vi "2P_AdapUprite_Linlin.vi"() -> ()   [LabVIEW 2015] (continued)
              frame True {
                n2515 = local read "wavelength(nm)"() -> (w5844:dbl)
                n2516 = call "pockelscellcalibration.vi"("l"=w5844, "T"=w5845) -> ("Vout"=w5843:dbl)
                n2517 = call "configuration_2P_Linlin.vi"("command"="get") -> ("config out"=w5841:T14)  [unwired: 2 in, 1 out]
                n2518 = Unbundle By Name(w5841) -> ("Vto2P"=w5848:i32, "AOlines"=w5847:tag[])
                n2519 = local write "Vpockels"(w5843) -> ()
                n2520 = property on="Laserpower  (%)" class="Slide (strict)"("Value"=w5845) -> ()  [unwired: 2 in, 2 out]
                n2521 = Index Array(array=w5847, index=w5848) -> (element=w5846:tag)
                n2522 = call-poly <vilib>:"DAQmx Create Virtual Channel.vi"("physical channels"=w5846) -> ("task out"=w5850:refnum<k21>, "error out"=w5849:errorcluster)  [unwired: 13 in]
                n2523 = call-poly <vilib>:"DAQmx Write.vi"("task/channels in"=w5850, "data"=w5843, "error in"=w5849) -> ("task out"=w5851:refnum<k21>, "error out"=w5852:errorcluster)  [unwired: 10 in, 1 out]
                n2524 = call <vilib>:"DAQmx Start Task.vi"("task/channels in"=w5851, "error in"=w5852) -> ("task out"=w5853:refnum<k21>, "error out"=w5854:errorcluster)  [unwired: 12 in]
                n2525 = call <vilib>:"DAQmx Stop Task.vi"("task/channels in"=w5853, "error in"=w5854) -> ("task out"=w5855:refnum<k21>, "error out"=w5856:errorcluster)  [unwired: 12 in]
                n2526 = call <vilib>:"DAQmx Clear Task.vi"("task in"=w5855, "error in"=w5856) -> ()  [unwired: 13 in, 1 out]
              }
            }
          }
          event "sealtest": Value Change {
            n2527 = event-data() -> ()  [unwired: 1 in, 6 out]
            n2528 = case shown="True" "sealtest" {
              frame False {
              }
              frame True {
                n2529 = stacked-sequence {
                  seq-local: [w5858 _ _ _ _ _ _] -> [_ w5893 _ w5945 _ _ _]
                  frame #0 {
                    n2530 = stacked-sequence {
                      tunnel: [_ w5872 _] -> w5858
                      frame #0 {
                        n2531 = call "2pparameters.vi"("command"="get") -> ("params out"=w5864:T12)  [unwired: 1 in]
                        n2532 = Unbundle By Name(w5864) -> ("autoshutter"=w5865:bool, "aAS"=w5859:u32[])
                        n2533 = local read "OCchecked?"() -> (w5862:bool)
                        n2534 = call "sealtestwfparams.vi"("command"="set") -> ()  [unwired: 6 in, 1 out]
                        n2535 = case shown="False" w5862 {
                          frame False {
                            n2536 = One Button Dialog(message="Is the OC gain correct?", button name ("OK")="ok") -> (true=w5866:bool)
                            n2537 = local write "OCchecked?"(w5866) -> ()
                          }
                          frame True {
                          }
                        }
                        n2538 = case shown="True" w5865 {
                          tunnel: w5859 -> [_ w5869]
                          frame False {
                          }
                          frame True {
                            n2539 = call "shuttercontrol_multi.vi"("Autoshutter Chans"=w5869, "command"="close") -> ()  [unwired: 1 in, 1 out]
                          }
                        }
                        n2540 = call "allAI-temp.vi"("command"=enum16{"get", "set", "clear", "append"}."clear") -> ()  [unwired: 3 in, 2 out]
                      }
                      frame #1 {
                        n2541 = call "sealtestwfparams.vi"("command"="get") -> ("Params out"=w5878:T25)  [unwired: 6 in]
                        n2542 = Unbundle By Name(w5878) -> ("AO parameters"=w5876:T26)
                        n2543 = Index Array(array=w5876, index=0) -> (element=w5875:T27)
                        n2544 = call "generateRampedSquareWave_fromAOparameters.vi"("AO params"=w5875) -> ("Waveform"=w5871:waveform(dbl), "wflength"=w5872:i32)
                        n2545 = Build Array(w5871) -> (w5874:waveform(dbl)[])
                        n2546 = call "waveformssealtestbuffer.vi"("AO wf in"=w5874, "command"="set") -> ()  [unwired: 1 out]
                      }
                      frame #2 {
                        n2547 = local read "Vholding (mV)"() -> (w5881:sgl)
                        n2548 = local read "Current Clamp"() -> (w5887:bool)
                        n2549 = local read "Voltage Clamp"() -> (w5886:bool)
                        n2550 = local read "OCgain"() -> (w5882:sgl)
                        n2551 = local read "CC_ICgain"() -> (w5885:dbl)
                        n2552 = local read "holdon"() -> (w5880:bool)
                        n2553 = call "patchparameters.vi"("command"="get") -> ("Params out"=w5889:T16)  [unwired: 1 in]
                        n2554 = Bundle By Name(cluster=w5889, "VC"=w5886, "CC"=w5887, "CC_icg (pA/mv)"=w5885, "VC_icg (mV/mV)"=10.0, "OCG (mV/pA)"=w5882, "OVG (mV/mV)"=0.1, "Vhold (mV)"=w5881, "holdon"=w5880) -> (w5888:T16)
                        n2555 = call "patchparameters.vi"("Params in"=w5888, "command"="set") -> ()  [unwired: 1 out]
                      }
                    }
                  }
                  frame #1 {
                    w5892 = 2
                    n2556 = call "patchparameters.vi"("command"="get") -> ("Params out"=w5900:T16)  [unwired: 1 in]
                    n2557 = Unbundle By Name(w5900) -> ("holdon"=w5899:bool, "Vhold (mV)"=w5898:sgl, "CC_icg (pA/mv)"=w5906:sgl, "CC"=w5904:bool, "VC_icg (mV/mV)"=w5905:sgl)
                    n2558 = Select(t=w5906, s=w5904, f=w5905) -> (s? t:f=w5907:sgl)
                    n2559 = To Single Precision Float(number=0.001 ("y")) -> (single precision float=w5908:sgl)
                    n2560 = Compound Arithmetic op=MULTIPLY(w5898, w5907, w5908) -> (w5902:sgl)
                    n2561 = case shown="False" w5899 {
                      tunnel: w5902 -> [_ w5920]
                      tunnel: [0.0 w5920] -> w5895
                      frame False {
                      }
                      frame True {
                      }
                    }
                    n2562 = Greater Than 0?(x=w5892) -> (x > 0?=w5894:bool)
                    n2563 = case shown="True" w5894 {
                      tunnel: w5893 -> [_ w5909]
                      tunnel: w5892 -> [_ w5912]
                      frame False {
                      }
                      frame True {
                        n2564 = Initialize Array(sgl 0.0 ("element"), w5912, w5909) -> (w5910:sgl[][])
                        n2565 = call "allAI-temp.vi"("array in"=w5910, "command"=enum16{"get", "set", "clear", "append"}."set") -> ()  [unwired: 2 in, 2 out]
                      }
                    }
                    n2566 = flat-sequence {
                      tunnel: w5893 -> [w5916]
                      tunnel: w5893 -> [w5915]
                      tunnel: [w5915] -> w5897
                      tunnel: [w5914] -> w5896
                      tunnel: w5895 -> [w5914]
                      tunnel: w5897 -> [w5918]
                      tunnel: w5896 -> [w5917]
                      frame #0 {
                        n2567 = call "prepAI_sealtest.vi"("samples per channel"=w5916) -> ()  [unwired: 2 in]
                      }
                      frame #1 {
                        n2568 = call "prepAO_sealtest.vi"("Vhold"=w5917, "samples per channel"=w5918) -> ()  [unwired: 1 in]
                      }
                    }
                  }
                  frame #2 {
                    n2569 = stacked-sequence {
                      frame #0 {
                        n2570 = call "tempconfigAO_seal.vi"("command"="get") -> ("Temp Config out"=w5924:T28)  [unwired: 1 in]
                        n2571 = Unbundle By Name(w5924) -> ("AO"=w5925:refnum<k21>[], "E_AO"=w5926:errorcluster[])
                        n2572 = for {
                          tunnel: w5925 -> [w5934] mode=indexing
                          tunnel: w5926 -> [w5933] mode=indexing
                          tunnel: [w5932] -> w5928 mode=indexing
                          tunnel: [w5931] -> w5929 mode=indexing
                          n2573 = call <vilib>:"DAQmx Start Task.vi"("task/channels in"=w5934, "error in"=w5933) -> ("task out"=w5932:refnum<k21>, "error out"=w5931:errorcluster)  [unwired: 12 in]
                        }
                        n2574 = call "tempconfigAO_seal.vi"("command"="get") -> ("Temp Config out"=w5927:T28)  [unwired: 1 in]
                        n2575 = Bundle By Name(cluster=w5927, "AO"=w5928, "E_AO"=w5929) -> (w5930:T28)
                        n2576 = call "tempconfigAO_seal.vi"("Temp Config in"=w5930, "command"="set") -> ()  [unwired: 1 out]
                      }
                      frame #1 {
                        n2577 = call "tempconfigAI_seal.vi"("command"="get") -> ("Temp Config out"=w5936:T29)  [unwired: 1 in]
                        n2578 = Unbundle By Name(w5936) -> ("AI"=w5941:refnum<k21>, "E_AI"=w5942:errorcluster)
                        n2579 = call <vilib>:"DAQmx Start Task.vi"("task/channels in"=w5941, "error in"=w5942) -> ("task out"=w5943:refnum<k21>, "error out"=w5944:errorcluster)  [unwired: 12 in]
                        n2580 = call "tempconfigAI_seal.vi"("command"="get") -> ("Temp Config out"=w5938:T29)  [unwired: 1 in]
                        n2581 = Bundle By Name(cluster=w5938, "AI"=w5943, "E_AI"=w5944) -> (w5940:T29)
                        n2582 = call "tempconfigAI_seal.vi"("Temp Config in"=w5940, "command"="set") -> ()  [unwired: 1 out]
                      }
                    }
                  }
                  frame #3 {
                    n2583 = while {
                      tunnel: w5945 -> [w5946]
                      stop <- w5947 stop-if-true
                      n2584 = stacked-sequence {
                        seq-local: [_ _ _ w5988 _ _] -> [_ _ _ _ w6040 _]
                        seq-local: [w5949 _ _ _ _ _] -> [_ w5958 _ w5981 w6029 w6060]
                        tunnel: w5946 -> [_ _ w5966 _ w6028 _]
                        frame #0 {
                          n2585 = call "patchparameters.vi"("command"="get") -> ("Params out"=w5956:T16)  [unwired: 1 in]
                          n2586 = local read "Vholding (mV)"() -> (w5953:sgl)
                          n2587 = Unbundle By Name(w5956) -> ("Vhold (mV)"=w5952:sgl, "holdon"=w5955:bool)
                          n2588 = local read "holdon"() -> (w5954:bool)
                          n2589 = Not Equal?(x=w5953, y=w5952) -> (x != y?=w5951:bool)
                          n2590 = Not Equal?(x=w5955, y=w5954) -> (x != y?=w5950:bool)
                          n2591 = Or(x=w5951, y=w5950) -> (x .or. y?=w5949:bool)
                        }
                        frame #1 {
                          n2592 = case shown="True" w5958 {
                            frame False {
                            }
                            frame True {
                              n2593 = local read "Vholding (mV)"() -> (w5961:sgl)
                              n2594 = local read "holdon"() -> (w5959:bool)
                              n2595 = call "patchparameters.vi"("command"="get") -> ("Params out"=w5962:T16)  [unwired: 1 in]
                              n2596 = Bundle By Name(cluster=w5962, "Vhold (mV)"=w5961, "holdon"=w5959) -> (w5960:T16)
                              n2597 = call "patchparameters.vi"("Params in"=w5960, "command"="set") -> ()  [unwired: 1 out]
                            }
                          }
                        }
                        frame #2 {
                          n2598 = call "tempconfigAI_seal.vi"("command"="get") -> ("Temp Config out"=w5976:T29)  [unwired: 1 in]
                          n2599 = Unbundle By Name(w5976) -> ("AI"=w5975:refnum<k21>, "E_AI"=w5974:errorcluster)
                          n2600 = call-poly <vilib>:"DAQmx Read.vi"("task/channels in"=w5975, "number of samples per channel"=w5966, "timeout"=10.0, "error in"=w5974) -> ("task out"=w5970:refnum<k21>, "data"=w5967:i16[][], "error out"=w5979:errorcluster)  [unwired: 9 in]
                          n2601 = call "tempconfigAI_seal.vi"("command"="get") -> ("Temp Config out"=w5971:T29)  [unwired: 1 in]
                          n2602 = Bundle By Name(cluster=w5971, "AI"=w5970, "E_AI"=w5979) -> (w5978:T29)
                          n2603 = To Single Precision Float(number=w5967) -> (single precision float=w5969:sgl[][])
                          n2604 = call "tempconfigAI_seal.vi"("Temp Config in"=w5978, "command"="set") -> ()  [unwired: 1 out]
                          n2605 = call "allAI-temp.vi"("array in"=w5969, "command"=enum16{"get", "set", "clear", "append"}."set") -> ()  [unwired: 2 in, 2 out]
                        }
                        frame #3 {
                          n2606 = case shown="True" w5981 {
                            frame False {
                            }
                            frame True {
                              n2607 = call "tempconfigAO_seal.vi"("command"="get") -> ("Temp Config out"=w6017:T28)  [unwired: 1 in]
                              n2608 = Unbundle By Name(w6017) -> ("AO"=w6016:refnum<k21>[], "E_AO"=w6015:errorcluster[])
                              n2609 = call "tempconfigAI_seal.vi"("command"="get") -> ("Temp Config out"=w6004:T29)  [unwired: 1 in]
                              n2610 = Unbundle By Name(w6004) -> ("AI"=w6005:refnum<k21>, "E_AI"=w6006:errorcluster)
                              n2611 = for {
                                tunnel: w6016 -> [w6021] mode=indexing
                                tunnel: w6015 -> [w6020] mode=indexing
                                tunnel: [w6019] -> w6011 mode=indexing
                                n2612 = call <vilib>:"DAQmx Stop Task.vi"("task/channels in"=w6021, "error in"=w6020) -> ("task out"=w6022:refnum<k21>, "error out"=w6023:errorcluster)  [unwired: 12 in]
                                n2613 = call <vilib>:"DAQmx Clear Task.vi"("task in"=w6022, "error in"=w6023) -> ("error out"=w6019:errorcluster)  [unwired: 13 in]
                              }
                              n2614 = call <vilib>:"DAQmx Stop Task.vi"("task/channels in"=w6005, "error in"=w6006) -> ("task out"=w6002:refnum<k21>, "error out"=w6001:errorcluster)  [unwired: 12 in]
                              n2615 = call <vilib>:"DAQmx Clear Task.vi"("task in"=w6002, "error in"=w6001) -> ("error out"=w6000:errorcluster)  [unwired: 13 in]
                              n2616 = call "tempconfigAO_seal.vi"("command"="get") -> ("Temp Config out"=w6012:T28)  [unwired: 1 in]
                              n2617 = Bundle By Name(cluster=w6012, "E_AO"=w6011) -> (w6010:T28)
                              n2618 = call "tempconfigAI_seal.vi"("command"="get") -> ("Temp Config out"=w6008:T29)  [unwired: 1 in]
                              n2619 = Bundle By Name(cluster=w6008, "E_AI"=w6000) -> (w5999:T29)
                              n2620 = call "tempconfigAO_seal.vi"("Temp Config in"=w6010, "command"="set") -> ()  [unwired: 1 out]
                              n2621 = call "tempconfigAI_seal.vi"("Temp Config in"=w5999, "command"="set") -> ()  [unwired: 1 out]
                            }
                          }
                          n2622 = call "allAI-temp.vi"("command"=enum16{"get", "set", "clear", "append"}."get") -> ("array out"=w5985:sgl[][])  [unwired: 3 in, 1 out]
                          n2623 = call "tempconfigAI_seal.vi"("command"="get") -> ("Temp Config out"=w5997:T29)  [unwired: 1 in]
                          n2624 = Unbundle By Name(w5997) -> ("header"=w5980:dbl[])
                          n2625 = Index Array(array=w5985, index (row) #1=1 ("index (row)"), index (row) #2=0 ("index (row)")) -> (element #1=w5983:sgl[], element #2=w5982:sgl[])  [unwired: 2 in]
                          n2626 = local read "OCgain"() -> (w5990:sgl)
                          n2627 = call "Unscaledtoscaled.vi"("Unscaled Data"=w5983, "Header Information"=w5980) -> ("Array"=w5995:sgl[])  [unwired: 1 in]
                          n2628 = call "Unscaledtoscaled.vi"("Unscaled Data"=w5982, "Header Information"=w5980) -> ("Array"=w5998:sgl[])  [unwired: 1 in]
                          n2629 = Multiply(x=w5995, y=0.1) -> (x*y=w5992:dbl[])
                          n2630 = Divide(x=w5998, y=w5990) -> (x/y=w5991:sgl[])
                          n2631 = Build Array(w5992, w5991) -> (w5994:dbl[][])
                          n2632 = Multiply(x=w5994, y=1000.0) -> (x*y=w5988:dbl[][])
                          "Patch readout" <- w5988
                        }
                        frame #4 {
                          n2633 = case shown="True" w6029 {
                            tunnel: w6028 -> [_ w6041]
                            frame False {
                            }
                            frame True {
                              n2634 = call "patchparameters.vi"("command"="get") -> ("Params out"=w6045:T16)  [unwired: 1 in]
                              n2635 = Unbundle By Name(w6045) -> ("holdon"=w6044:bool, "Vhold (mV)"=w6043:sgl, "CC_icg (pA/mv)"=w6051:sgl, "CC"=w6049:bool, "VC_icg (mV/mV)"=w6050:sgl)
                              n2636 = Select(t=w6051, s=w6049, f=w6050) -> (s? t:f=w6052:sgl)
                              n2637 = To Single Precision Float(number=0.001 ("y")) -> (single precision float=w6053:sgl)
                              n2638 = Compound Arithmetic op=MULTIPLY(w6043, w6052, w6053) -> (w6047:sgl)
                              n2639 = case shown="True" w6044 {
                                tunnel: w6047 -> [_ w6058]
                                tunnel: [0.0 w6058] -> w6042
                                frame False {
                                }
                                frame True {
                                }
                              }
                              n2640 = flat-sequence {
                                tunnel: w6041 -> [w6054]
                                tunnel: w6042 -> [w6056]
                                tunnel: w6041 -> [w6055]
                                frame #0 {
                                n2641 = call "prepAI_sealtest.vi"("samples per channel"=w6054) -> ()  [unwired: 2 in]
                                }
                                frame #1 {
                                n2642 = call "prepAO_sealtest.vi"("Vhold"=w6056, "samples per channel"=w6055) -> ()  [unwired: 1 in]
                                }
                              }
                            }
                          }
                          n2643 = call "sealtestwfparams.vi"("command"="get") -> ("Params out"=w6034:T25)  [unwired: 6 in]
                          n2644 = Unbundle By Name(w6034) -> ("AO parameters"=w6035:T26)
                          n2645 = Index Array(array=w6035, index=0) -> (element=w6037:T27)
                          n2646 = Unbundle By Name(w6037) -> ("Cycles"=w6032:dbl, "Start amplitude (V)"=w6031:dbl, "Sampling frequency (Hz)"=w6030:dbl)
                          n2647 = local read "fitpoints"() -> (w6038:dbl)
                          n2648 = script code="V=data(1,:);\nI=data(2,:);\ntres=mean(V);\nspc=(nsamp./ncyc);\nV=V(spc+1:end-spc);\nI=I(spc+1:end-spc);\ndV=mean(V(V>tres))-mean(V(V<tres))\nIcyc=reshape(I,[spc ncyc-2]);\nIcyc=Icyc';\nIcyc=mean(Icyc,1);\ndIss=mean(Icyc(floor(spc*0.15):floor(spc/2)-2))-mean(Icyc(spc*0.65:spc-2))\nRm=dV*1e3/dIss;\n[maxi,ind]=max(Icyc);\nIfit=Icyc(ind+1:ind+1+points-1)-0.5*(mean(Icyc(floor(spc*0.15):floor(spc/2)-2))+mean(Icyc(spc*0.65:spc-2)))\nt=(3:points-1+3)./srate*1000;\nt=t';\nIfit=Ifit';\nc=fit(t,Ifit, 'exp1');\ncoeffs=coeffvalues(c);\nIa=coeffs(1);\nRa=dV*1e3./Ia/2;\ntau=-1./coeffs(2);\ncap=tau/Ra*1000;"("data"=w6040, "nsamp"=w6028, "ncyc"=w6032, "maxV"=w6031, "points"=w6038, "srate"=w6030) -> ("cap"=w6027:dbl, "Ra"=w6026:dbl, "Icyc"=w6025:dbl[], "Rm"=w6024:dbl)  [unwired: 1 in, 1 out]
                          n2649 = local read "set as Rp?"() -> (w6039:bool)
                          n2650 = local write "Cmembrane"(w6027) -> ()
                          n2651 = local write "Rmembrane (MOhm)"(w6024) -> ()
                          n2652 = local write "Racces (MOhm)"(w6026) -> ()
                          n2653 = case shown="True" w6039 {
                            tunnel: w6024 -> [_ w6059]
                            frame False {
                            }
                            frame True {
                              n2654 = local write "Rpipette (MOhm)"(w6059) -> ()
                            }
                          }
                          n2655 = local write "Ifit"(w6025) -> ()
                        }
                        frame #5 {
                          n2656 = local read "set as Rp?"() -> (w6061:bool)
                          n2657 = case shown="True" w6060 {
                            frame False {
                            }
                            frame True {
                              n2658 = stacked-sequence {
                                frame #0 {
                                n2659 = call "tempconfigAO_seal.vi"("command"="get") -> ("Temp Config out"=w6068:T28)  [unwired: 1 in]
                                n2660 = Unbundle By Name(w6068) -> ("AO"=w6067:refnum<k21>[], "E_AO"=w6066:errorcluster[])
                                n2661 = for {
                                tunnel: w6067 -> [w6075] mode=indexing
                                tunnel: w6066 -> [w6074] mode=indexing
                                tunnel: [w6073] -> w6064 mode=indexing
                                tunnel: [w6072] -> w6063 mode=indexing
                                n2662 = call <vilib>:"DAQmx Start Task.vi"("task/channels in"=w6075, "error in"=w6074) -> ("task out"=w6073:refnum<k21>, "error out"=w6072:errorcluster)  [unwired: 12 in]
                                }
                                n2663 = call "tempconfigAO_seal.vi"("command"="get") -> ("Temp Config out"=w6065:T28)  [unwired: 1 in]
                                n2664 = Bundle By Name(cluster=w6065, "AO"=w6064, "E_AO"=w6063) -> (w6062:T28)
                                n2665 = call "tempconfigAO_seal.vi"("Temp Config in"=w6062, "command"="set") -> ()  [unwired: 1 out]
                                }
                                frame #1 {
                                n2666 = call "tempconfigAI_seal.vi"("command"="get") -> ("Temp Config out"=w6077:T29)  [unwired: 1 in]
                                n2667 = Unbundle By Name(w6077) -> ("AI"=w6082:refnum<k21>, "E_AI"=w6083:errorcluster)
                                n2668 = call <vilib>:"DAQmx Start Task.vi"("task/channels in"=w6082, "error in"=w6083) -> ("task out"=w6084:refnum<k21>, "error out"=w6085:errorcluster)  [unwired: 12 in]
                                n2669 = call "tempconfigAI_seal.vi"("command"="get") -> ("Temp Config out"=w6079:T29)  [unwired: 1 in]
                                n2670 = Bundle By Name(cluster=w6079, "AI"=w6084, "E_AI"=w6085) -> (w6081:T29)
                                n2671 = call "tempconfigAI_seal.vi"("Temp Config in"=w6081, "command"="set") -> ()  [unwired: 1 out]
                                }
                              }
                            }
                          }
                          n2672 = case shown="True" w6061 {
                            frame False {
                            }
                            frame True {
                              n2673 = local write "set as Rp?"(FALSE ("set as Rp?")) -> ()
                            }
                          }
                        }
                      }
                      n2674 = local read "sealtest"() -> (w5948:bool)
                      n2675 = Not(x=w5948) -> (.not. x?=w5947:bool)
                    }
                  }
                  frame #4 {
                    n2676 = call "tempconfigAO_seal.vi"("command"="get") -> ("Temp Config out"=w6112:T28)  [unwired: 1 in]
                    n2677 = call "configuration_2P_Linlin.vi"("command"="get") -> ("config out"=w6087:T14)  [unwired: 2 in, 1 out]
                    n2678 = Unbundle By Name(w6112) -> ("AO"=w6111:refnum<k21>[], "E_AO"=w6110:errorcluster[])
                    n2679 = call "tempconfigAI_seal.vi"("command"="get") -> ("Temp Config out"=w6099:T29)  [unwired: 1 in]
                    n2680 = Unbundle By Name(w6099) -> ("AI"=w6100:refnum<k21>, "E_AI"=w6101:errorcluster)
                    n2681 = Unbundle By Name(w6087) -> ("Device 1 sampleclock out"=w6092:tag, "Device 1 Starttrigger out"=w6091:tag)
                    n2682 = for {
                      tunnel: w6111 -> [w6116] mode=indexing
                      tunnel: w6110 -> [w6115] mode=indexing
                      tunnel: [w6114] -> w6106 mode=indexing
                      n2683 = call <vilib>:"DAQmx Stop Task.vi"("task/channels in"=w6116, "error in"=w6115) -> ("task out"=w6117:refnum<k21>, "error out"=w6118:errorcluster)  [unwired: 12 in]
                      n2684 = call <vilib>:"DAQmx Clear Task.vi"("task in"=w6117, "error in"=w6118) -> ("error out"=w6114:errorcluster)  [unwired: 13 in]
                    }
                    n2685 = call <vilib>:"DAQmx Stop Task.vi"("task/channels in"=w6100, "error in"=w6101) -> ("task out"=w6097:refnum<k21>, "error out"=w6096:errorcluster)  [unwired: 12 in]
                    n2686 = call <vilib>:"DAQmx Disconnect Terminals.vi"("source terminal"=tag "/Dev1/ai/SampleClock", "destination terminal"=w6092) -> ("error out"=w6089:errorcluster)  [unwired: 13 in]
                    n2687 = call <vilib>:"DAQmx Clear Task.vi"("task in"=w6097, "error in"=w6096) -> ("error out"=w6095:errorcluster)  [unwired: 13 in]
                    n2688 = call "tempconfigAO_seal.vi"("command"="get") -> ("Temp Config out"=w6107:T28)  [unwired: 1 in]
                    n2689 = Bundle By Name(cluster=w6107, "E_AO"=w6106) -> (w6105:T28)
                    n2690 = call "tempconfigAI_seal.vi"("command"="get") -> ("Temp Config out"=w6103:T29)  [unwired: 1 in]
                    n2691 = Bundle By Name(cluster=w6103, "E_AI"=w6095) -> (w6094:T29)
                    n2692 = call "tempconfigAO_seal.vi"("Temp Config in"=w6105, "command"="set") -> ()  [unwired: 1 out]
                    n2693 = call "tempconfigAI_seal.vi"("Temp Config in"=w6094, "command"="set") -> ()  [unwired: 1 out]
                    n2694 = call <vilib>:"DAQmx Disconnect Terminals.vi"("source terminal"=tag "/Dev1/ai/StartTrigger", "destination terminal"=w6091, "error in"=w6089) -> ()  [unwired: 12 in, 1 out]
                  }
                  frame #5 {
                    n2695 = call "zeropatch.vi"() -> ()  [unwired: 12 in]
                  }
                  frame #6 {
                    w6122 = T24 4 items=["no dialog", "OK message", "continue or stop message", "OK message + warnings", "continue/stop + warnings"] ("type of dialog (OK msg:1)")
                    n2696 = call "displayerrors.vi"() -> ("error IO"=w6121:errorcluster)
                    n2697 = call <vilib>:"Simple Error Handler.vi"("type of dialog (OK msg:1)"=w6122, "error in (no error)"=w6121) -> ("error out"=w6120:errorcluster)  [unwired: 3 in, 4 out]
                    n2698 = call <vilib>:"Clear Errors.vi"("error in (no error)"=w6120) -> ("error out"=w6119:errorcluster)  [unwired: 5 in, 1 out]
                    n2699 = call "seterrors.vi"("error IO"=w6119) -> ()
                  }
                }
              }
            }
          }
          event "readpatch": Value Change {
            n2700 = event-data() -> ()  [unwired: 1 in, 6 out]
            n2701 = local read "readpatch"() -> (w6123:bool)
            n2702 = case shown="True" w6123 {
              frame False {
              }
              frame True {
                n2703 = stacked-sequence {
                  seq-local: [w6124 _ _ _ _ _] -> [_ w6159 _ w6211 _ _]
                  frame #0 {
                    n2704 = stacked-sequence {
                      tunnel: [_ w6138 _] -> w6124
                      frame #0 {
                        n2705 = call "2pparameters.vi"("command"="get") -> ("params out"=w6130:T12)  [unwired: 1 in]
                        n2706 = Unbundle By Name(w6130) -> ("autoshutter"=w6131:bool, "aAS"=w6125:u32[])
                        n2707 = local read "OCchecked?"() -> (w6128:bool)
                        n2708 = call "sealtestwfparams.vi"("command"="set") -> ()  [unwired: 6 in, 1 out]
                        n2709 = case shown="False" w6128 {
                          frame False {
                            n2710 = One Button Dialog(message="Is the OC gain correct?", button name ("OK")="ok") -> (true=w6132:bool)
                            n2711 = local write "OCchecked?"(w6132) -> ()
                          }
                          frame True {
                          }
                        }
                        n2712 = case shown="True" w6131 {
                          tunnel: w6125 -> [_ w6135]
                          frame False {
                          }
                          frame True {
                            n2713 = call "shuttercontrol_multi.vi"("Autoshutter Chans"=w6135, "command"="close") -> ()  [unwired: 1 in, 1 out]
                          }
                        }
                        n2714 = call "allAI-temp.vi"("command"=enum16{"get", "set", "clear", "append"}."clear") -> ()  [unwired: 3 in, 2 out]
                      }
                      frame #1 {
                        n2715 = call "sealtestwfparams.vi"("command"="get") -> ("Params out"=w6144:T25)  [unwired: 6 in]
                        n2716 = Unbundle By Name(w6144) -> ("AO parameters"=w6142:T26)
                        n2717 = Index Array(array=w6142, index=1) -> (element=w6141:T27)
                        n2718 = call "generateRampedSquareWave_fromAOparameters.vi"("AO params"=w6141) -> ("Waveform"=w6137:waveform(dbl), "wflength"=w6138:i32)
                        n2719 = Build Array(w6137) -> (w6140:waveform(dbl)[])
                        n2720 = call "waveformssealtestbuffer.vi"("AO wf in"=w6140, "command"="set") -> ()  [unwired: 1 out]
                      }
                      frame #2 {
                        n2721 = local read "Vholding (mV)"() -> (w6147:sgl)
                        n2722 = local read "Current Clamp"() -> (w6153:bool)
                        n2723 = local read "Voltage Clamp"() -> (w6152:bool)
                        n2724 = local read "OCgain"() -> (w6148:sgl)
                        n2725 = local read "CC_ICgain"() -> (w6151:dbl)
                        n2726 = local read "holdon"() -> (w6146:bool)
                        n2727 = call "patchparameters.vi"("command"="get") -> ("Params out"=w6155:T16)  [unwired: 1 in]
                        n2728 = Bundle By Name(cluster=w6155, "VC"=w6152, "CC"=w6153, "CC_icg (pA/mv)"=w6151, "VC_icg (mV/mV)"=10.0, "OCG (mV/pA)"=w6148, "OVG (mV/mV)"=0.1, "Vhold (mV)"=w6147, "holdon"=w6146) -> (w6154:T16)
                        n2729 = call "patchparameters.vi"("Params in"=w6154, "command"="set") -> ()  [unwired: 1 out]
                      }
                    }
                  }
                  frame #1 {
                    w6158 = 2
                    n2730 = call "patchparameters.vi"("command"="get") -> ("Params out"=w6166:T16)  [unwired: 1 in]
                    n2731 = Unbundle By Name(w6166) -> ("holdon"=w6165:bool, "Vhold (mV)"=w6164:sgl, "CC_icg (pA/mv)"=w6172:sgl, "CC"=w6170:bool, "VC_icg (mV/mV)"=w6171:sgl)
                    n2732 = Select(t=w6172, s=w6170, f=w6171) -> (s? t:f=w6173:sgl)
                    n2733 = To Single Precision Float(number=0.001 ("y")) -> (single precision float=w6174:sgl)
                    n2734 = Compound Arithmetic op=MULTIPLY(w6164, w6173, w6174) -> (w6168:sgl)
                    n2735 = case shown="False" w6165 {
                      tunnel: w6168 -> [_ w6186]
                      tunnel: [0.0 w6186] -> w6161
                      frame False {
                      }
                      frame True {
                      }
                    }
                    n2736 = Greater Than 0?(x=w6158) -> (x > 0?=w6160:bool)
                    n2737 = case shown="True" w6160 {
                      tunnel: w6159 -> [_ w6175]
                      tunnel: w6158 -> [_ w6178]
                      frame False {
                      }
                      frame True {
                        n2738 = Initialize Array(sgl 0.0 ("element"), w6178, w6175) -> (w6176:sgl[][])
                        n2739 = call "allAI-temp.vi"("array in"=w6176, "command"=enum16{"get", "set", "clear", "append"}."set") -> ()  [unwired: 2 in, 2 out]
                      }
                    }
                    n2740 = flat-sequence {
                      tunnel: w6159 -> [w6182]
                      tunnel: w6159 -> [w6181]
                      tunnel: [w6181] -> w6163
                      tunnel: [w6180] -> w6162
                      tunnel: w6161 -> [w6180]
                      tunnel: w6163 -> [w6184]
                      tunnel: w6162 -> [w6183]
                      frame #0 {
                        n2741 = call "prepAI_sealtest.vi"("samples per channel"=w6182) -> ()  [unwired: 2 in]
                      }
                      frame #1 {
                        n2742 = call "prepAO_sealtest.vi"("Vhold"=w6183, "samples per channel"=w6184) -> ()  [unwired: 1 in]
                      }
                    }
                  }
                  frame #2 {
                    n2743 = stacked-sequence {
                      frame #0 {
                        n2744 = call "tempconfigAO.vi"("command"="get") -> ("Temp Config out"=w6190:T28)  [unwired: 1 in]
                        n2745 = Unbundle By Name(w6190) -> ("AO"=w6191:refnum<k21>[], "E_AO"=w6192:errorcluster[])
                        n2746 = for {
                          tunnel: w6191 -> [w6200] mode=indexing
                          tunnel: w6192 -> [w6199] mode=indexing
                          tunnel: [w6198] -> w6194 mode=indexing
                          tunnel: [w6197] -> w6195 mode=indexing
                          n2747 = call <vilib>:"DAQmx Start Task.vi"("task/channels in"=w6200, "error in"=w6199) -> ("task out"=w6198:refnum<k21>, "error out"=w6197:errorcluster)  [unwired: 12 in]
                        }
                        n2748 = call "tempconfigAO.vi"("command"="get") -> ("Temp Config out"=w6193:T28)  [unwired: 1 in]
                        n2749 = Bundle By Name(cluster=w6193, "AO"=w6194, "E_AO"=w6195) -> (w6196:T28)
                        n2750 = call "tempconfigAO.vi"("Temp Config in"=w6196, "command"="set") -> ()  [unwired: 1 out]
                      }
                      frame #1 {
                        n2751 = call "tempconfigAI.vi"("command"="get") -> ("Temp Config out"=w6202:T29)  [unwired: 1 in]
                        n2752 = Unbundle By Name(w6202) -> ("AI"=w6207:refnum<k21>, "E_AI"=w6208:errorcluster)
                        n2753 = call <vilib>:"DAQmx Start Task.vi"("task/channels in"=w6207, "error in"=w6208) -> ("task out"=w6209:refnum<k21>, "error out"=w6210:errorcluster)  [unwired: 12 in]
                        n2754 = call "tempconfigAI.vi"("command"="get") -> ("Temp Config out"=w6204:T29)  [unwired: 1 in]
                        n2755 = Bundle By Name(cluster=w6204, "AI"=w6209, "E_AI"=w6210) -> (w6206:T29)
                        n2756 = call "tempconfigAI.vi"("Temp Config in"=w6206, "command"="set") -> ()  [unwired: 1 out]
                      }
                    }
                  }
                  frame #3 {
                    n2757 = while {
                      tunnel: w6211 -> [w6212]
                      stop <- w6213 stop-if-true
                      n2758 = local read "readpatch"() -> (w6216:bool)
                      n2759 = Not(x=w6216) -> (.not. x?=w6215:bool)
                      n2760 = case shown="False" w6215 {
                        tunnel: w6212 -> [w6217 _]
                        frame False {
                          n2761 = stacked-sequence {
                            seq-local: [w6218 _ _ _ _ _] -> [_ w6227 _ w6250 w6297 w6316]
                            tunnel: w6217 -> [_ _ w6235 _ w6296 _]
                            frame #0 {
                              n2762 = call "patchparameters.vi"("command"="get") -> ("Params out"=w6225:T16)  [unwired: 1 in]
                              n2763 = local read "Vholding (mV)"() -> (w6222:sgl)
                              n2764 = Unbundle By Name(w6225) -> ("Vhold (mV)"=w6221:sgl, "holdon"=w6224:bool)
                              n2765 = local read "holdon"() -> (w6223:bool)
                              n2766 = Not Equal?(x=w6222, y=w6221) -> (x != y?=w6220:bool)
                              n2767 = Not Equal?(x=w6224, y=w6223) -> (x != y?=w6219:bool)
                              n2768 = Or(x=w6220, y=w6219) -> (x .or. y?=w6218:bool)
                            }
                            frame #1 {
                              n2769 = case shown="False" w6227 {
                                frame False {
                                }
                                frame True {
                                n2770 = local read "Vholding (mV)"() -> (w6230:sgl)
                                n2771 = local read "holdon"() -> (w6228:bool)
                                n2772 = call "patchparameters.vi"("command"="get") -> ("Params out"=w6231:T16)  [unwired: 1 in]
                                n2773 = Bundle By Name(cluster=w6231, "Vhold (mV)"=w6230, "holdon"=w6228) -> (w6229:T16)
                                n2774 = call "patchparameters.vi"("Params in"=w6229, "command"="set") -> ()  [unwired: 1 out]
                                }
                              }
                            }
                            frame #2 {
                              n2775 = call "tempconfigAI.vi"("command"="get") -> ("Temp Config out"=w6245:T29)  [unwired: 1 in]
                              n2776 = Unbundle By Name(w6245) -> ("AI"=w6244:refnum<k21>, "E_AI"=w6243:errorcluster)
                              n2777 = call-poly <vilib>:"DAQmx Read.vi"("task/channels in"=w6244, "number of samples per channel"=w6235, "timeout"=10.0, "error in"=w6243) -> ("task out"=w6239:refnum<k21>, "data"=w6236:i16[][], "error out"=w6248:errorcluster)  [unwired: 9 in]
                              n2778 = call "tempconfigAI.vi"("command"="get") -> ("Temp Config out"=w6240:T29)  [unwired: 1 in]
                              n2779 = Bundle By Name(cluster=w6240, "AI"=w6239, "E_AI"=w6248) -> (w6247:T29)
                              n2780 = To Single Precision Float(number=w6236) -> (single precision float=w6238:sgl[][])
                              n2781 = call "tempconfigAI.vi"("Temp Config in"=w6247, "command"="set") -> ()  [unwired: 1 out]
                              n2782 = call "allAI-temp.vi"("array in"=w6238, "command"=enum16{"get", "set", "clear", "append"}."set") -> ()  [unwired: 2 in, 2 out]
                            }
                            frame #3 {
                              n2783 = case shown="True" w6250 {
                                frame False {
                                }
                                frame True {
                                n2784 = call "tempconfigAO.vi"("command"="get") -> ("Temp Config out"=w6289:T28)  [unwired: 1 in]
                                n2785 = Unbundle By Name(w6289) -> ("AO"=w6288:refnum<k21>[], "E_AO"=w6287:errorcluster[])
                                n2786 = call "tempconfigAI.vi"("command"="get") -> ("Temp Config out"=w6276:T29)  [unwired: 1 in]
                                n2787 = Unbundle By Name(w6276) -> ("AI"=w6277:refnum<k21>, "E_AI"=w6278:errorcluster)
                                n2788 = for {
                                tunnel: w6288 -> [w6293] mode=indexing
                                tunnel: w6287 -> [w6292] mode=indexing
                                tunnel: [w6291] -> w6283 mode=indexing
                                n2789 = call <vilib>:"DAQmx Stop Task.vi"("task/channels in"=w6293, "error in"=w6292) -> ("task out"=w6294:refnum<k21>, "error out"=w6295:errorcluster)  [unwired: 12 in]
                                n2790 = call <vilib>:"DAQmx Clear Task.vi"("task in"=w6294, "error in"=w6295) -> ("error out"=w6291:errorcluster)  [unwired: 13 in]
                                }
                                n2791 = call <vilib>:"DAQmx Stop Task.vi"("task/channels in"=w6277, "error in"=w6278) -> ("task out"=w6274:refnum<k21>, "error out"=w6273:errorcluster)  [unwired: 12 in]
                                n2792 = call <vilib>:"DAQmx Clear Task.vi"("task in"=w6274, "error in"=w6273) -> ("error out"=w6272:errorcluster)  [unwired: 13 in]
                                n2793 = call "tempconfigAO.vi"("command"="get") -> ("Temp Config out"=w6284:T28)  [unwired: 1 in]
                                n2794 = Bundle By Name(cluster=w6284, "E_AO"=w6283) -> (w6282:T28)
                                n2795 = call "tempconfigAI.vi"("command"="get") -> ("Temp Config out"=w6280:T29)  [unwired: 1 in]
                                n2796 = Bundle By Name(cluster=w6280, "E_AI"=w6272) -> (w6271:T29)
                                n2797 = call "tempconfigAO.vi"("Temp Config in"=w6282, "command"="set") -> ()  [unwired: 1 out]
                                n2798 = call "tempconfigAI.vi"("Temp Config in"=w6271, "command"="set") -> ()  [unwired: 1 out]
                                }
                              }
                              n2799 = call "allAI-temp.vi"("command"=enum16{"get", "set", "clear", "append"}."get") -> ("array out"=w6254:sgl[][])  [unwired: 3 in, 1 out]
                              n2800 = call "tempconfigAI.vi"("command"="get") -> ("Temp Config out"=w6266:T29)  [unwired: 1 in]
                              n2801 = call "tempconfigAI.vi"("command"="get") -> ("Temp Config out"=w6268:T29)  [unwired: 1 in]
                              n2802 = Unbundle By Name(w6266) -> ("header"=w6264:dbl[])
                              n2803 = Unbundle By Name(w6268) -> ("header"=w6270:dbl[])
                              n2804 = Index Array(array=w6254, index (row) #1=1 ("index (row)"), index (row) #2=0 ("index (row)")) -> (element #1=w6252:sgl[], element #2=w6251:sgl[])  [unwired: 2 in]
                              n2805 = local read "OCgain"() -> (w6258:sgl)
                              n2806 = call "Unscaledtoscaled.vi"("Unscaled Data"=w6252, "Header Information"=w6264) -> ("Array"=w6263:sgl[])  [unwired: 1 in]
                              n2807 = call "Unscaledtoscaled.vi"("Unscaled Data"=w6251, "Header Information"=w6270) -> ("Array"=w6267:sgl[])  [unwired: 1 in]
                              n2808 = Multiply(x=w6263, y=0.1) -> (x*y=w6260:dbl[])
                              n2809 = Divide(x=w6267, y=w6258) -> (x/y=w6259:sgl[])
                              n2810 = Build Array(w6260, w6259) -> (w6262:dbl[][])
                              n2811 = Multiply(x=w6262, y=1000.0) -> (x*y=w6249:dbl[][])
                              n2812 = local write "Patch readout"(w6249) -> ()
                            }
                            frame #4 {
                              n2813 = case shown="True" w6297 {
                                tunnel: w6296 -> [_ w6298]
                                frame False {
                                }
                                frame True {
                                n2814 = call "patchparameters.vi"("command"="get") -> ("Params out"=w6302:T16)  [unwired: 1 in]
                                n2815 = Unbundle By Name(w6302) -> ("holdon"=w6301:bool, "Vhold (mV)"=w6300:sgl, "CC_icg (pA/mv)"=w6308:sgl, "CC"=w6306:bool, "VC_icg (mV/mV)"=w6307:sgl)
                                n2816 = Select(t=w6308, s=w6306, f=w6307) -> (s? t:f=w6309:sgl)
                                n2817 = To Single Precision Float(number=0.001 ("y")) -> (single precision float=w6310:sgl)
                                n2818 = Compound Arithmetic op=MULTIPLY(w6300, w6309, w6310) -> (w6304:sgl)
                                n2819 = case shown="True" w6301 {
                                tunnel: w6304 -> [_ w6315]
                                tunnel: [0.0 w6315] -> w6299
                                frame False {
                                }
                                frame True {
                                }
                                }
                                n2820 = flat-sequence {
                                tunnel: w6298 -> [w6311]
                                tunnel: w6299 -> [w6313]
                                tunnel: w6298 -> [w6312]
                                frame #0 {
                                n2821 = call "prepAI_sealtest.vi"("samples per channel"=w6311) -> ()  [unwired: 2 in]
                                }
                                frame #1 {
                                n2822 = call "prepAO_sealtest.vi"("Vhold"=w6313, "samples per channel"=w6312) -> ()  [unwired: 1 in]
                                }
                                }
                                }
                              }
                            }
                            frame #5 {
                              n2823 = case shown="True" w6316 {
                                frame False {
                                }
                                frame True {
                                n2824 = stacked-sequence {
                                frame #0 {
                                n2825 = call "tempconfigAO.vi"("command"="get") -> ("Temp Config out"=w6323:T28)  [unwired: 1 in]
                                n2826 = Unbundle By Name(w6323) -> ("AO"=w6322:refnum<k21>[], "E_AO"=w6321:errorcluster[])
                                n2827 = for {
                                tunnel: w6322 -> [w6330] mode=indexing
                                tunnel: w6321 -> [w6329] mode=indexing
                                tunnel: [w6328] -> w6319 mode=indexing
                                tunnel: [w6327] -> w6318 mode=indexing
                                n2828 = call <vilib>:"DAQmx Start Task.vi"("task/channels in"=w6330, "error in"=w6329) -> ("task out"=w6328:refnum<k21>, "error out"=w6327:errorcluster)  [unwired: 12 in]
                                }
                                n2829 = call "tempconfigAO.vi"("command"="get") -> ("Temp Config out"=w6320:T28)  [unwired: 1 in]
                                n2830 = Bundle By Name(cluster=w6320, "AO"=w6319, "E_AO"=w6318) -> (w6317:T28)
                                n2831 = call "tempconfigAO.vi"("Temp Config in"=w6317, "command"="set") -> ()  [unwired: 1 out]
                                }
                                frame #1 {
                                n2832 = call "tempconfigAI.vi"("command"="get") -> ("Temp Config out"=w6332:T29)  [unwired: 1 in]
                                n2833 = Unbundle By Name(w6332) -> ("AI"=w6337:refnum<k21>, "E_AI"=w6338:errorcluster)
                                n2834 = call <vilib>:"DAQmx Start Task.vi"("task/channels in"=w6337, "error in"=w6338) -> ("task out"=w6339:refnum<k21>, "error out"=w6340:errorcluster)  [unwired: 12 in]
                                n2835 = call "tempconfigAI.vi"("command"="get") -> ("Temp Config out"=w6334:T29)  [unwired: 1 in]
                                n2836 = Bundle By Name(cluster=w6334, "AI"=w6339, "E_AI"=w6340) -> (w6336:T29)
                                n2837 = call "tempconfigAI.vi"("Temp Config in"=w6336, "command"="set") -> ()  [unwired: 1 out]
                                }
                                }
                                }
                              }
                            }
                          }
                        }
                        frame True {
                        }
                      }
                      n2838 = local read "readpatch"() -> (w6214:bool)
                      n2839 = Not(x=w6214) -> (.not. x?=w6213:bool)
                    }
                  }
                  frame #4 {
                    n2840 = call "tempconfigAO.vi"("command"="get") -> ("Temp Config out"=w6366:T28)  [unwired: 1 in]
                    n2841 = call "configuration_2P_Linlin.vi"("command"="get") -> ("config out"=w6342:T14)  [unwired: 2 in, 1 out]
                    n2842 = Unbundle By Name(w6366) -> ("AO"=w6365:refnum<k21>[], "E_AO"=w6364:errorcluster[])
                    n2843 = call "tempconfigAI.vi"("command"="get") -> ("Temp Config out"=w6353:T29)  [unwired: 1 in]
                    n2844 = Unbundle By Name(w6342) -> ("Device 1 sampleclock out"=w6346:tag, "Device 1 Starttrigger out"=w6345:tag)
                    n2845 = Unbundle By Name(w6353) -> ("AI"=w6354:refnum<k21>, "E_AI"=w6355:errorcluster)
                    n2846 = for {
                      tunnel: w6365 -> [w6370] mode=indexing
                      tunnel: w6364 -> [w6369] mode=indexing
                      tunnel: [w6368] -> w6360 mode=indexing
                      n2847 = call <vilib>:"DAQmx Stop Task.vi"("task/channels in"=w6370, "error in"=w6369) -> ("task out"=w6371:refnum<k21>, "error out"=w6372:errorcluster)  [unwired: 12 in]
                      n2848 = call <vilib>:"DAQmx Clear Task.vi"("task in"=w6371, "error in"=w6372) -> ("error out"=w6368:errorcluster)  [unwired: 13 in]
                    }
                    n2849 = call <vilib>:"DAQmx Stop Task.vi"("task/channels in"=w6354, "error in"=w6355) -> ("task out"=w6351:refnum<k21>, "error out"=w6350:errorcluster)  [unwired: 12 in]
                    n2850 = call <vilib>:"DAQmx Disconnect Terminals.vi"("source terminal"=tag "/Dev1/ai/SampleClock", "destination terminal"=w6346) -> ("error out"=w6343:errorcluster)  [unwired: 13 in]
                    n2851 = call <vilib>:"DAQmx Clear Task.vi"("task in"=w6351, "error in"=w6350) -> ("error out"=w6349:errorcluster)  [unwired: 13 in]
                    n2852 = call "tempconfigAO.vi"("command"="get") -> ("Temp Config out"=w6361:T28)  [unwired: 1 in]
                    n2853 = Bundle By Name(cluster=w6361, "E_AO"=w6360) -> (w6359:T28)
                    n2854 = call "tempconfigAI.vi"("command"="get") -> ("Temp Config out"=w6357:T29)  [unwired: 1 in]
                    n2855 = Bundle By Name(cluster=w6357, "E_AI"=w6349) -> (w6348:T29)
                    n2856 = call "tempconfigAO.vi"("Temp Config in"=w6359, "command"="set") -> ()  [unwired: 1 out]
                    n2857 = call <vilib>:"DAQmx Disconnect Terminals.vi"("source terminal"=tag "/Dev1/ai/StartTrigger", "destination terminal"=w6345, "error in"=w6343) -> ()  [unwired: 12 in, 1 out]
                    n2858 = call "tempconfigAI.vi"("Temp Config in"=w6348, "command"="set") -> ()  [unwired: 1 out]
                  }
                  frame #5 {
                    w6375 = T24 4 items=["no dialog", "OK message", "continue or stop message", "OK message + warnings", "continue/stop + warnings"] ("type of dialog (OK msg:1)")
                    n2859 = call "displayerrors.vi"() -> ("error IO"=w6374:errorcluster)
                    n2860 = call "zeropatch.vi"() -> ()  [unwired: 12 in]
                    n2861 = call <vilib>:"Simple Error Handler.vi"("type of dialog (OK msg:1)"=w6375, "error in (no error)"=w6374) -> ("error out"=w6373:errorcluster)  [unwired: 3 in, 4 out]
                    n2862 = call <vilib>:"Clear Errors.vi"("error in (no error)"=w6373) -> ()  [unwired: 5 in, 2 out]
                  }
                }
              }
            }
          }
          event "Current Clamp": Value Change {
            n2863 = event-data() -> ()  [unwired: 1 in, 6 out]
            n2864 = local read "Current Clamp"() -> (w6380:bool)
            n2865 = property on="Vholding (mV)" class="DigNum (strict)"("Caption.Text"="Ihold (pA)") -> ()  [unwired: 2 in, 2 out]
            n2866 = Not(x=w6380) -> (.not. x?=w6379:bool)
            n2867 = property on="Voltage Clamp" class="Bool (strict)"("Value"=w6379) -> ()  [unwired: 2 in, 2 out]
            n2868 = One Button Dialog(message="Have you switched the HEKA to CC and changed the external input cable?", button name ("OK")="Ok") -> ()  [unwired: 1 out]
          }
          event "Voltage Clamp": Value Change {
            n2869 = event-data() -> ()  [unwired: 1 in, 6 out]
            n2870 = local read "Voltage Clamp"() -> (w6385:bool)
            n2871 = Not(x=w6385) -> (.not. x?=w6384:bool)
            n2872 = property on="Current Clamp" class="Bool (strict)"("Value"=w6384) -> ()  [unwired: 2 in, 2 out]
            n2873 = One Button Dialog(message="Have you switched the HEKA to VC and changed the external input cable?", button name ("OK")="Ok") -> ()  [unwired: 1 out]
            n2874 = property on="Vholding (mV)" class="DigNum (strict)"("Caption.Text"="Vhold (mV)") -> ()  [unwired: 2 in, 2 out]
          }
          event "OCgain": Value Change {
            n2875 = event-data() -> ()  [unwired: 1 in, 6 out]
            n2876 = local read "OCgain"() -> (w6388:sgl)
            n2877 = Less?(x=w6388, y=0.3) -> (x < y?=w6386:bool)
            n2878 = case shown="True" w6386 {
              frame False {
                w6389 = 10.0 items=["0.1"=10.0, "10"=0.1] ("CC_ICgain")
                n2879 = local write "CC_ICgain"(w6389) -> ()
              }
              frame True {
                w6390 = 0.1 items=["0.1"=10.0, "10"=0.1] ("CC_ICgain")
                n2880 = local write "CC_ICgain"(w6390) -> ()
              }
            }
          }
          event "holdon": Value Change {
            n2881 = event-data() -> ()  [unwired: 1 in, 6 out]
            n2882 = stacked-sequence {
              frame #0 {
                n2883 = local read "Vholding (mV)"() -> (w6394:sgl)
                n2884 = local read "holdon"() -> (w6391:bool)
                n2885 = call "patchparameters.vi"("command"="get") -> ("Params out"=w6395:T16)  [unwired: 1 in]
                n2886 = Bundle By Name(cluster=w6395, "Vhold (mV)"=w6394, "holdon"=w6391) -> (w6392:T16)
                n2887 = call "patchparameters.vi"("Params in"=w6392, "command"="set") -> ()  [unwired: 1 out]
              }
              frame #1 {
                n2888 = call "zeropatch.vi"() -> ()  [unwired: 12 in]
              }
            }
          }
          event "Vholding (mV)": Value Change {
            n2889 = event-data() -> ()  [unwired: 1 in, 6 out]
            n2890 = local read "holdon"() -> (w6397:bool)
            n2891 = case shown="True" w6397 {
              frame False {
              }
              frame True {
                n2892 = stacked-sequence {
                  frame #0 {
                    n2893 = local read "Vholding (mV)"() -> (w6400:sgl)
                    n2894 = local read "holdon"() -> (w6401:bool)
                    n2895 = call "patchparameters.vi"("command"="get") -> ("Params out"=w6402:T16)  [unwired: 1 in]
                    n2896 = Bundle By Name(cluster=w6402, "Vhold (mV)"=w6400, "holdon"=w6401) -> (w6398:T16)
                    n2897 = call "patchparameters.vi"("Params in"=w6398, "command"="set") -> ()  [unwired: 1 out]
                  }
                  frame #1 {
                    n2898 = call "zeropatch.vi"() -> ()  [unwired: 12 in]
                  }
                }
              }
            }
          }
          event "AI channels": Value Change {
            n2899 = event-data() -> ()  [unwired: 1 in, 6 out]
            n2900 = local read "CI channels"() -> (w6411:i32[])
            n2901 = local read "AI channels"() -> (w6412:i32[])
            n2902 = call "configuration_2P_Linlin.vi"("command"="get") -> ("config out"=w6405:T14)  [unwired: 2 in, 1 out]
            n2903 = Unbundle By Name(w6405) -> ("CI names"=w6407:string[], "AI names"=w6408:string[])
            n2904 = for {
              tunnel: w6411 -> [w6417] mode=indexing
              tunnel: w6407 -> [w6418]
              tunnel: [w6416] -> w6409 mode=indexing
              n2905 = Index Array(array=w6418, index=w6417) -> (element=w6416:string)
            }
            n2906 = for {
              tunnel: w6412 -> [w6414] mode=indexing
              tunnel: w6408 -> [w6415]
              tunnel: [w6413] -> w6410 mode=indexing
              n2907 = Index Array(array=w6415, index=w6414) -> (element=w6413:string)
            }
            n2908 = Build Array (concatenate)(w6409, w6410) -> (w6406:string[])
            n2909 = property on="image1list" class="Ring (strict)"("Strings []"=w6406) -> ()  [unwired: 2 in, 2 out]
            n2910 = property on="image2list" class="Ring (strict)"("Strings []"=w6406) -> ()  [unwired: 2 in, 2 out]
            n2911 = property on="image1list chA" class="Ring (strict)"("Strings []"=w6406) -> ()  [unwired: 2 in, 2 out]
            n2912 = property on="image1list chB" class="Ring (strict)"("Strings []"=w6406) -> ()  [unwired: 2 in, 2 out]
          }
          event "CI channels": Value Change {
            n2913 = event-data() -> ()  [unwired: 1 in, 6 out]
            n2914 = local read "CI channels"() -> (w6426:i32[])
            n2915 = local read "AI channels"() -> (w6427:i32[])
            n2916 = call "configuration_2P_Linlin.vi"("command"="get") -> ("config out"=w6419:T14)  [unwired: 2 in, 1 out]
            n2917 = Unbundle By Name(w6419) -> ("CI names"=w6422:string[], "AI names"=w6423:string[])
            n2918 = for {
              tunnel: w6426 -> [w6432] mode=indexing
              tunnel: w6422 -> [w6433]
              tunnel: [w6431] -> w6424 mode=indexing
              n2919 = Index Array(array=w6433, index=w6432) -> (element=w6431:string)
            }
            n2920 = for {
              tunnel: w6427 -> [w6429] mode=indexing
              tunnel: w6423 -> [w6430]
              tunnel: [w6428] -> w6425 mode=indexing
              n2921 = Index Array(array=w6430, index=w6429) -> (element=w6428:string)
            }
            n2922 = Build Array (concatenate)(w6424, w6425) -> (w6421:string[])
            n2923 = property on="image1list" class="Ring (strict)"("Strings []"=w6421) -> ()  [unwired: 2 in, 2 out]
            n2924 = property on="image2list" class="Ring (strict)"("Strings []"=w6421) -> ()  [unwired: 2 in, 2 out]
            n2925 = property on="image1list chA" class="Ring (strict)"("Strings []"=w6421) -> ()  [unwired: 2 in, 2 out]
            n2926 = property on="image1list chB" class="Ring (strict)"("Strings []"=w6421) -> ()  [unwired: 2 in, 2 out]
          }
          event "setdatdir": Value Change {
            n2927 = event-data() -> ()  [unwired: 1 in, 5 out]
            n2928 = case shown="True" "setdatdir" {
              frame False {
              }
              frame True {
                n2929 = stacked-sequence {
                  frame #0 {
                    n2930 = local read "data dir"() -> (w6435:path)
                    n2931 = call "File Dialog"("start path"=w6435, "prompt"="Please select data directory...") -> ("selected path"=w6437:path, "cancelled"=w6436:bool, "error out"=w6438:errorcluster)  [unwired: 10 in, 1 out]
                    n2932 = case shown="False" w6436 {
                      tunnel: w6437 -> [w6448 _]
                      tunnel: w6438 -> [w6446 w6449]
                      tunnel: [w6441 w6449] -> w6440
                      frame False {
                        n2933 = local write "data dir"(w6448) -> ()
                        n2934 = call "configuration_2P_Linlin.vi"("error in"=w6446, "command"="get") -> ("Error out"=w6442:errorcluster, "config out"=w6445:T14)  [unwired: 1 in]
                        n2935 = Bundle By Name(cluster=w6445, "master data dir"=w6448) -> (w6443:T14)
                        n2936 = call "configuration_2P_Linlin.vi"("error in"=w6442, "config in"=w6443, "command"="set") -> ("Error out"=w6441:errorcluster)  [unwired: 1 out]
                      }
                      frame True {
                      }
                    }
                    n2937 = local write "status"(w6440) -> ()
                  }
                  frame #1 {
                    n2938 = property on="setdatdir" class="Bool (strict)"("Value"=FALSE ("setdatdir")) -> ()  [unwired: 2 in, 2 out]
                  }
                }
              }
            }
          }
          event "Shutter": Value Change {
            n2939 = event-data() -> ()  [unwired: 1 in, 5 out]
            n2940 = local read "Auto Shutter Channels"() -> (w6451:i32[])
            n2941 = case shown="True" "Shutter" {
              tunnel: w6451 -> [w6453 w6455]
              frame False {
                n2942 = call "shuttercontrol_multi.vi"("Autoshutter Chans"=w6453, "command"="close") -> ()  [unwired: 1 in, 1 out]
              }
              frame True {
                n2943 = call "shuttercontrol_multi.vi"("Autoshutter Chans"=w6455, "command"="open") -> ()  [unwired: 1 in, 1 out]
              }
            }
          }
          event "ROI": Value Change {
            n2944 = event-data() -> ()  [unwired: 1 in, 5 out]
            n2945 = local read "ROI"() -> (w6457:bool)
            n2946 = case shown="True" w6457 {
              frame False {
              }
              frame True {
                n2947 = stacked-sequence {
                  frame #0 {
                    n2948 = local read "Square pixels"() -> (w6474:bool)
                    n2949 = local read "square matrix"() -> (w6473:bool)
                    n2950 = local read "Vx-max ref"() -> (w6479:dbl)
                    n2951 = local read "Vx-min ref"() -> (w6478:dbl)
                    n2952 = local read "Vy-min ref"() -> (w6475:dbl)
                    n2953 = local read "ypixels ref"() -> (w6477:i32)
                    n2954 = local read "Vy-max ref"() -> (w6476:dbl)
                    n2955 = local read "xpixels ref"() -> (w6480:i32)
                    n2956 = local read "Angle ref"() -> (w6472:dbl)
                    n2957 = local read "Colormap"() -> (w6481:i32)
                    n2958 = call "2pparameters.vi"("command"="get") -> ("params out"=w6484:T12)  [unwired: 1 in]
                    n2959 = Bundle By Name(cluster=w6484, "Xpixels Img"=w6480, "Vx-min Img"=w6478, "VX-max Img"=w6479, "Ypixels Img"=w6477, "Vy-min Img"=w6475, "Vy-max Img"=w6476, "Colormap"=w6481, "square pixels"=w6474, "square matrix"=w6473, "Angle Img"=w6472) -> (w6483:T12)
                    n2960 = call "2pparameters.vi"("Params in"=w6483, "command"="set") -> ()  [unwired: 1 out]
                    n2961 = local read "Vx-max draw"() -> (w6464:dbl)
                    n2962 = local read "Angle drawing"() -> (w6471:dbl)
                    n2963 = local read "Vx-min draw"() -> (w6465:dbl)
                    n2964 = local read "Vy-min draw"() -> (w6468:dbl)
                    n2965 = local read "ypixels draw"() -> (w6466:dbl)
                    n2966 = local read "Vy-max draw"() -> (w6467:dbl)
                    n2967 = local read "Square pixels"() -> (w6469:bool)
                    n2968 = local read "square matrix"() -> (w6470:bool)
                    n2969 = local read "xpixels draw"() -> (w6463:dbl)
                    n2970 = local read "Colormap"() -> (w6462:i32)
                    n2971 = call "2pparameters.vi"("command"="get") -> ("params out"=w6459:T12)  [unwired: 1 in]
                    n2972 = Bundle By Name(cluster=w6459, "Xpixels"=w6463, "Vxminref"=w6465, "Vxmaxref"=w6464, "Ypixels"=w6466, "Vyminref"=w6468, "Vymaxref"=w6467, "Colormap"=w6462, "square pixels"=w6469, "square matrix"=w6470, "Angle draw"=w6471) -> (w6460:T12)
                    n2973 = call "2pparameters.vi"("Params in"=w6460, "command"="set") -> ()  [unwired: 1 out]
                  }
                  frame #1 {
                    n2974 = Current VI's Path() -> (path=w6495:path)
                    n2975 = Strip Path(path=w6495) -> (stripped path=w6496:path)  [unwired: 1 out]
                    n2976 = Build Path(base path=w6496, name or relative path="subVIs\\Image\\SetROI_v4.vi") -> (appended path=w6494:path)
                    n2977 = call <vilib>:"Set Busy.vi"() -> ("error out"=w6492:errorcluster)  [unwired: 10 in, 1 out]
